vi "Set Meta Data (Serial Ref).vi"(7 "meta data":T1[](array[typedef]), 8 "error in":errorcluster, 11 "VISA resource name":refnum<visa-resource-name>) -> (0 "error out":errorcluster, 3 "connection info out":T2)   [LabVIEW 2010, in "NI STM.lvlib"]
doc: "Assigns the meta data cluster associated with this STM session."
uses:
  NI STM.lvlib
  Serial Connection Info.ctl
  SubVIs/MetaDataElement.ctl
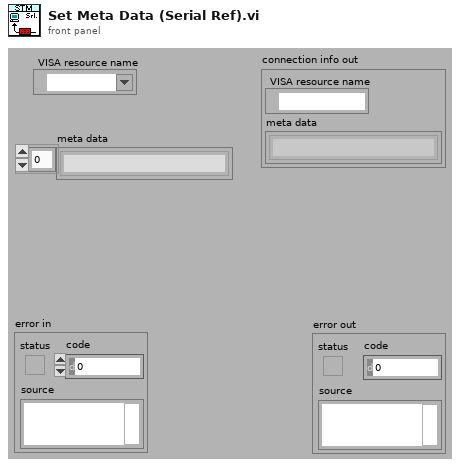
[diagram p1: front panel]
types:
  T1 = typedef "NI STM.lvlib/MetaDataElement.ctl" = string
  T2 = typedef "NI STM.lvlib/Serial Connection Info.ctl" = cluster{"VISA resource name":refnum<visa-resource-name>, "meta data":T1[]}
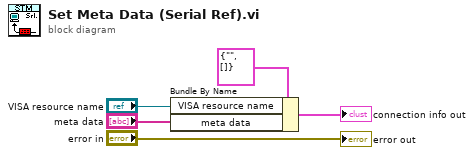
[diagram p0: block diagram]
diagram:
  n1 = Bundle By Name(cluster=T2 {"VISA resource name"="", "meta data"=[]} ("Connection Info"), "VISA resource name"="VISA resource name", "meta data"="meta data") -> (→"connection info out":T2)
  "error out" <- "error in"
